vi "gen_i0X_data.vi"(0 "Raw Image Data In":T3, 7 "Processed Image Data In":T4, 11 "Input data":T1) -> (4 "Raw Image Data Out":T3, 8 "Processed Image Data In Out":T4, 12 "A Counts":u32, 14 "B Counts":u32)   [LabVIEW 2023]
uses:
  <vilib>/vision/Image Controls.llb/IMAQ Image.ctl
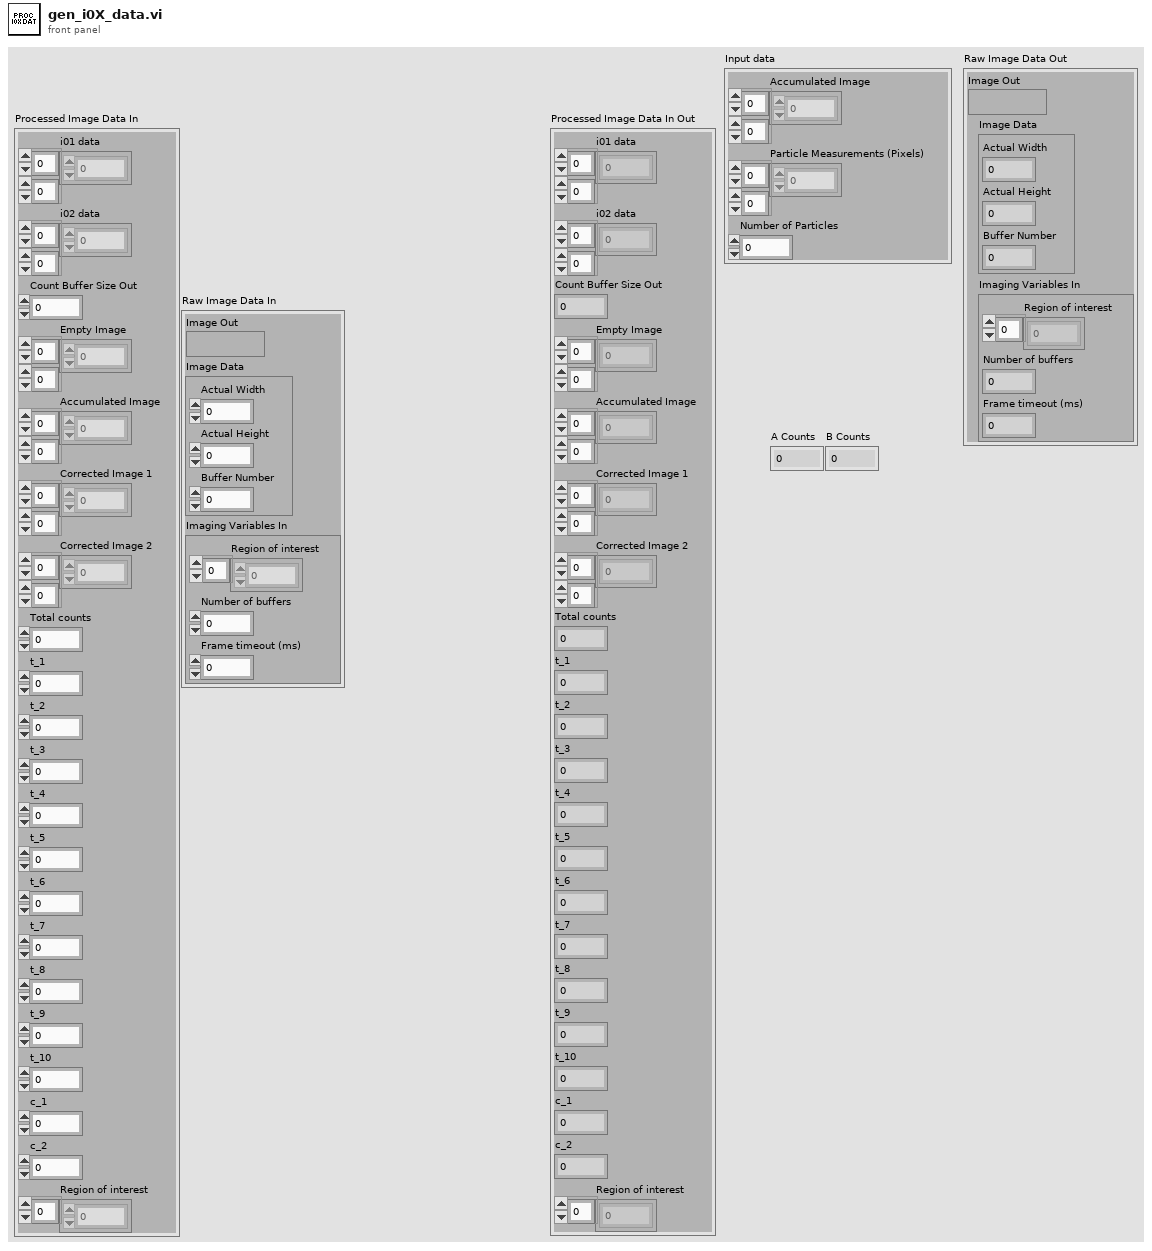
[diagram p1: front panel]
types:
  T1 = cluster{"Accumulated Image":i16[][], "Particle Measurements (Pixels)":dbl[][], "Number of Particles":u16}
  T2 = typedef "IMAQ Image.ctl" = refnum<image>
  T3 = cluster{"Image Out":T2, "Image Data":cluster{"Actual Width":u32, "Actual Height":u32, "Buffer Number":i32}, "Imaging Variables In":cluster{"Region of interest":i32[], "Number of buffers":u32, "Frame timeout (ms)":u32}}
  T4 = cluster{"i01 data":sgl[][], "i02 data":sgl[][], "Count Buffer Size Out":i32, "Empty Image":i16[][], "Accumulated Image":i16[][], "Corrected Image 1":i16[][], "Corrected Image 2":i16[][], "Total counts":i32, "t_1":i32, "t_2":i32, "t_3":i32, "t_4":i32, "t_5":i32, "t_6":i32, "t_7":i32, "t_8":i32, "t_9":i32, "t_10":i32, "c_1":i32, "c_2":i32, "Region of interest":i32[]}
  T5 = cluster{"Actual Width":u32, "Actual Height":u32, "Buffer Number":i32}
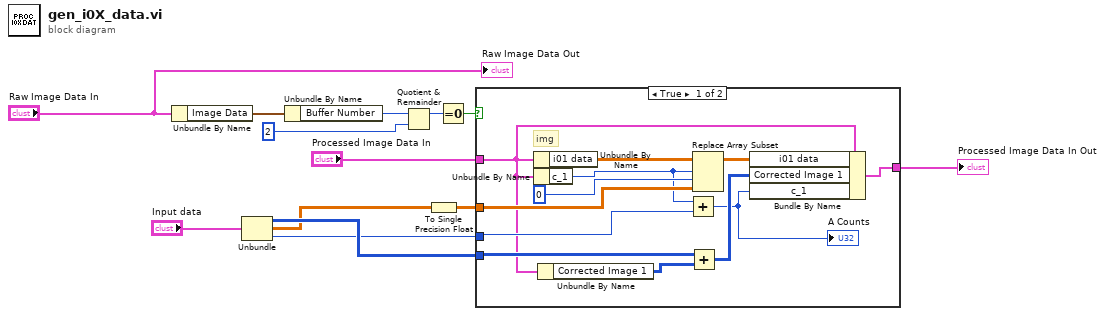
[diagram p0: block diagram]
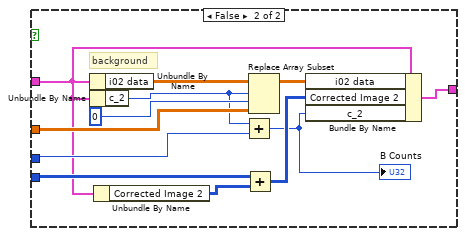
[diagram p2: hidden frame]
diagram:
  n1 = Unbundle By Name("Raw Image Data In") -> ("Image Data"=w6:T5)
  n2 = Unbundle("Input data") -> ("Accumulated Image"=w4:i16[][], "Particle Measurements (Pixels)"=w3:dbl[][], "Number of Particles"=w2:u16)
  n3 = Unbundle By Name(w6) -> ("Buffer Number"=w12:i32)
  n4 = Quotient & Remainder(x=w12, y=2) -> (x-y*floor(x/y)=w11:i32)  [unwired: 1 out]
  n5 = To Single Precision Float(number=w3) -> (single precision float=w10:sgl[][])
  n6 = Equal To 0?(x=w11) -> (x = 0?=w13:bool)
  n7 = case shown="True" w13 {
    tunnel: "Processed Image Data In" -> [w17 w29]
    tunnel: w10 -> [w23 w35]
    tunnel: w2 -> [w20 w32]
    tunnel: w4 -> [w19 w31]
    tunnel: [w15 w27] -> w8
    frame True {
      # "img"
      n8 = Unbundle By Name(w17) -> ("i01 data"=w25:sgl[][])
      n9 = Unbundle By Name(w17) -> ("c_1"=w21:i32)
      n10 = Unbundle By Name(w17) -> ("Corrected Image 1"=w18:i16[][])
      n11 = Add(x=w21, y=w20) -> (x+y=w14:i32)
      "A Counts" <- w14
      n12 = Add(x=w19, y=w18) -> (x+y=w16:i16[][])
      n13 = Replace Array Subset(array=w25, new element=w23, index (row)=w21, index (col)=0 ("disabled index (col)")) -> (w22:sgl[][])
      n14 = Bundle By Name(cluster=w17, "i01 data"=w22, "Corrected Image 1"=w16, "c_1"=w14) -> (w15:T4)
    }
    frame False {
      # "background"
      n15 = Unbundle By Name(w29) -> ("i02 data"=w37:sgl[][])
      n16 = Unbundle By Name(w29) -> ("c_2"=w33:i32)
      n17 = Unbundle By Name(w29) -> ("Corrected Image 2"=w30:i16[][])
      n18 = Add(x=w33, y=w32) -> (x+y=w26:i32)
      "B Counts" <- w26
      n19 = Add(x=w31, y=w30) -> (x+y=w28:i16[][])
      n20 = Replace Array Subset(array=w37, new element=w35, index (row)=w33, index (col)=0 ("disabled index (col)")) -> (w34:sgl[][])
      n21 = Bundle By Name(cluster=w29, "i02 data"=w34, "Corrected Image 2"=w28, "c_2"=w26) -> (w27:T4)
    }
  }
  "Processed Image Data In Out" <- w8
  "Raw Image Data Out" <- "Raw Image Data In"
